vi "DebAddLog.vi"(0 "Type":i32, 1 "Log":i32[](array[numeric]), 2 "Time":i32, 4 "Error":i32, 5 "error in":errorcluster) -> (19 "error out":errorcluster)   [LabVIEW 2018]
uses:
  DebCommandLog.vi
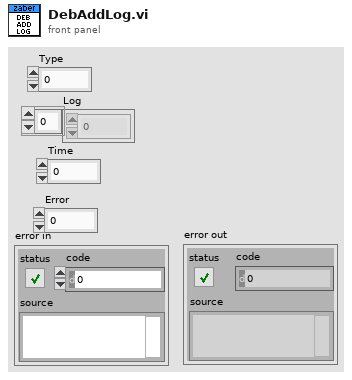
[diagram p1: front panel]
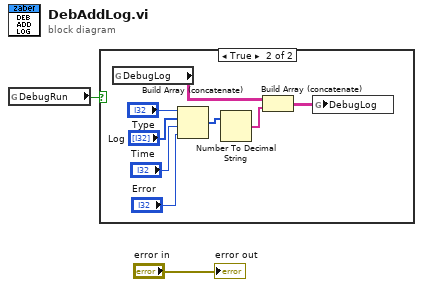
[diagram p0: block diagram]
diagram:
  n1 = global read "DebCommandLog.vi" "DebugRun"() -> (w1:bool)
  n2 = case shown="True" w1 {
    frame False {
    }
    frame True {
      n3 = global read "DebCommandLog.vi" "DebugLog"() -> (w10:string[][])
      n4 = Build Array (concatenate)("Type", "Log", "Time", "Error") -> (w5:i32[])
      n5 = Number To Decimal String(number=w5) -> (decimal integer string=w4:string[])  [unwired: 1 in]
      n6 = Build Array (concatenate)(w10, w4) -> (w9:string[][])
      n7 = global write "DebCommandLog.vi" "DebugLog"(w9) -> ()
    }
  }
  "error out" <- "error in"
